vi "CI_Gnl_SetFillColor.vi"(8 "error in":errorcluster, 10 "Value":u8, 11 "Display State In":T1={"StandardColor"=15671808, "WarningColor"=15671808, "CriticalColor"=15671808, "Standard<>Warning Range"=0, "Warning<>Critical Range"=0} caption="State") -> (0 "error out":errorcluster, 3 "FillColor":u32(colorbox)=15671808)   [LabVIEW 2010, in "CapacityIndicator.xctl"]
doc: "Copyright 2007 SAPHIR (Olivier JOURDAN) All Rights Reserved\n\nThis VI return appropriate color according to the slide value."
uses:
  CapacityIndicator.xctl
  CI_State.ctl
panel:
  # "Input"
  # "Output"
  # "Local"
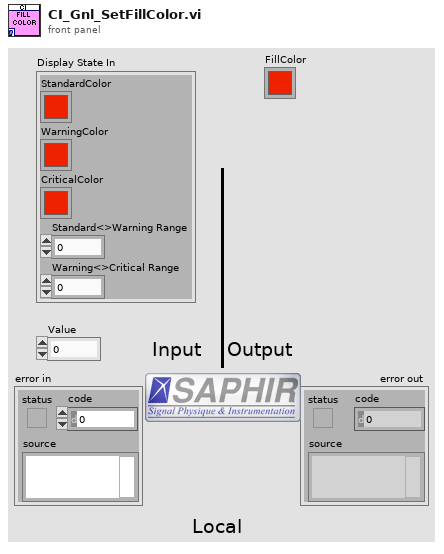
[diagram p1: front panel]
types:
  T1 = typedef "CapacityIndicator.xctl/CI_State.ctl" = cluster{"StandardColor":u32, "WarningColor":u32, "CriticalColor":u32, "Standard<>Warning Range":u8, "Warning<>Critical Range":u8}
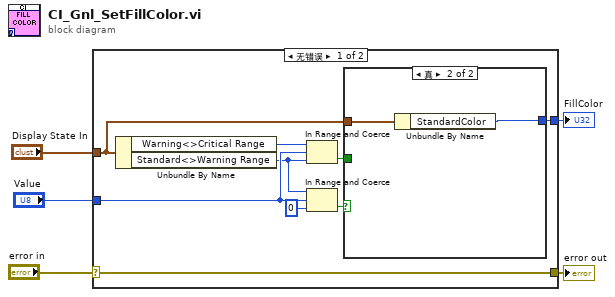
[diagram p0: block diagram]
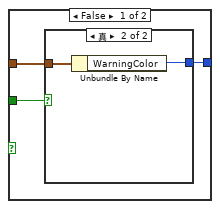
[diagram p2: hidden frame]
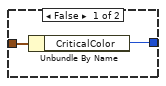
[diagram p3: hidden frame]
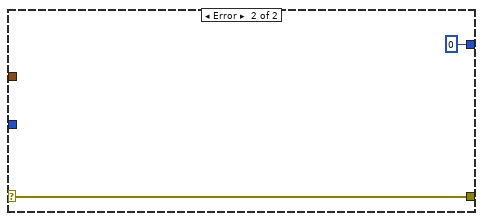
[diagram p4: hidden frame]
diagram:
  n1 = case shown="无错误" "error in" {
    selector: "error in" -> [w6 w25]
    tunnel: "Value" -> [w13 _]
    tunnel: "Display State In" -> [w9 _]
    tunnel: [w7 u32 0 ("StandardColor")] -> w3
    tunnel: [w6 w25] -> w1
    frame No Error {
      n2 = Unbundle By Name(w9) -> ("Warning<>Critical Range"=w11:u8, "Standard<>Warning Range"=w12:u8)
      n3 = In Range and Coerce(upper limit=w11, x=w13, lower limit=w12) -> (In Range?=w8:bool)  [unwired: 1 out]
      n4 = In Range and Coerce(upper limit=w12, x=w13, lower limit=u8 0) -> (In Range?=w10:bool)  [unwired: 1 out]
      n5 = case shown="真" w10 {
        tunnel: w9 -> [w17 w23]
        tunnel: w8 -> [w15 _]
        tunnel: [w16 w22] -> w7
        frame False {
          n6 = case shown="真" w15 {
            tunnel: w17 -> [w19 w21]
            tunnel: [w18 w20] -> w16
            frame False {
              n7 = Unbundle By Name(w19) -> ("CriticalColor"=w18:u32)
            }
            frame True {
              n8 = Unbundle By Name(w21) -> ("WarningColor"=w20:u32)
            }
          }
        }
        frame True {
          n9 = Unbundle By Name(w23) -> ("StandardColor"=w22:u32)
        }
      }
    }
    frame Error {
    }
  }
  "FillColor" <- w3
  "error out" <- w1
